vi "Table Controls.vi"() -> ()   [LabVIEW 2013, in "DCAF UI Elements.lvlib"]
uses:
  Controls/DCAF UI Elements.lvlib
  Controls/Add.ctl
  Controls/Configure.ctl
  Controls/Remove.ctl
panel:
  in  "Remove":T1
  in  "Configure":T2
  in  "Add":T3
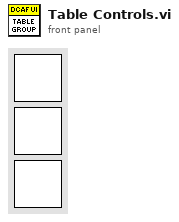
[diagram p1: front panel]
types:
  T1 = typedef "DCAF UI Elements.lvlib/Remove.ctl" = bool
  T2 = typedef "DCAF UI Elements.lvlib/Configure.ctl" = bool
  T3 = typedef "DCAF UI Elements.lvlib/Add.ctl" = bool
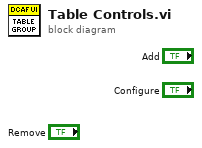
[diagram p0: block diagram]
diagram:
